vi "Run.vi"(8 "error in (no error)":errorcluster) -> (0 "error out":errorcluster)   [LabVIEW 2017, in "loggingModule.lvlib"]
uses:
  loggingModule.lvlib
  UEFGV/Type Def/UEFGV_States.ctl
  TypeDefs/LoopStates.ctl
  Queue/TypeDefs/queueFGVState.ctl
  ErrorMonitor/ErrorMonitor.lvlib
panel:
  out "stop":bool
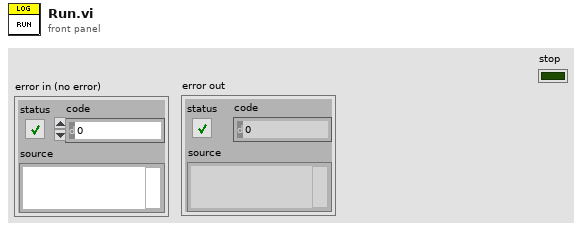
[diagram p1: front panel]
types:
  T1 = typedef "UEFGV_States.ctl" = enum16{"Create", "Get", "Destroy"}
  T2 = enum16{"open", "replace", "create", "open or create", "replace or create", "replace or create with confirmation"}
  T3 = typedef "LoopStates.ctl" = enum16{"start", "wait", "run", "end"}
  T4 = typedef "loggingModule.lvlib/queueFGVState.ctl" = enum16{"obtain", "enqueue low priority", "enqueue high priority", "dequeue", "release"}
  T5 = typedef "loggingModule.lvlib/message.ctl" = cluster{"calling module":string, "message":string, "data":variant}
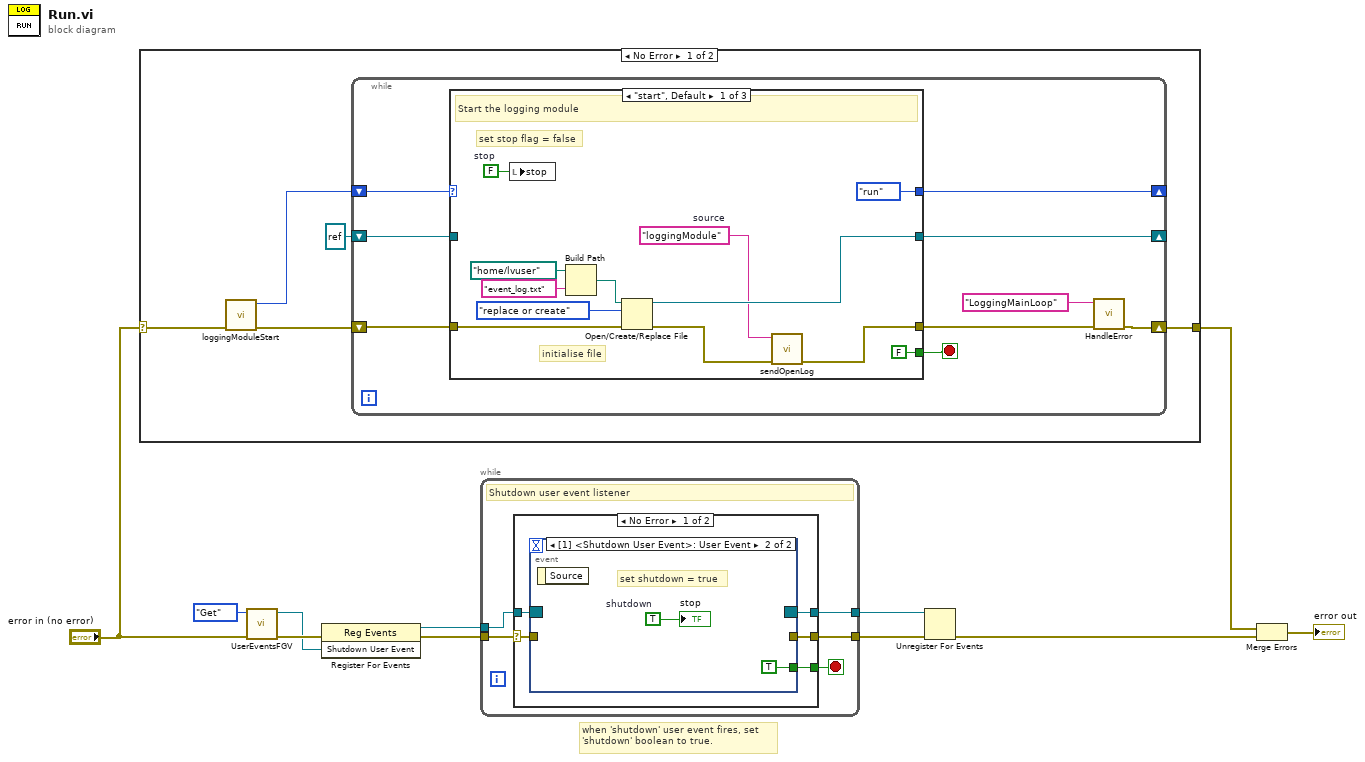
[diagram p0: block diagram]
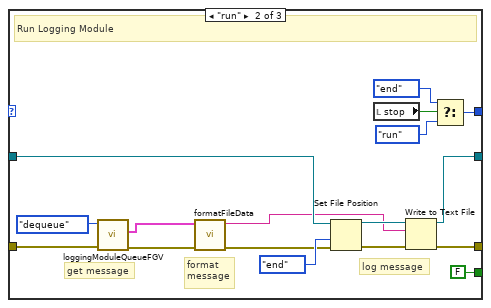
[diagram p2: hidden frame]
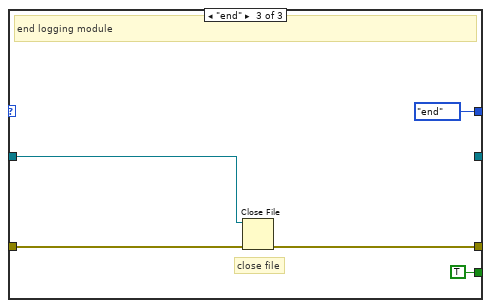
[diagram p3: hidden frame]
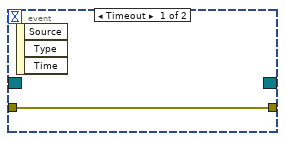
[diagram p5: hidden frame]
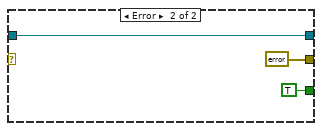
[diagram p6: hidden frame]
diagram:
  # "when 'shutdown' user event fires, set\n'shutdown' boolean to true."
  n1 = case shown="No Error" "error in (no error)" {
    selector: "error in (no error)" -> [w16 w60]
    tunnel: [w12 w60] -> w3
    frame No Error {
      n2 = call "loggingModuleStart.vi"("error in (no error)"=w16) -> ("error out"=w14:errorcluster, "message out"=w15:T3)  [unwired: 9 in]
      n3 = while {
        shift-right: [w23] -> _
        shift-left: w15 -> [w25]
        shift-right: [w17] -> w12
        shift-left: w14 -> [w22]
        shift-right: [w21] -> _
        shift-left: refnum<file> refnum ("refnum out") -> [w20]
        stop <- w24 stop-if-true
        n4 = case shown="\"start\", Default" w25 {
          tunnel: [FALSE FALSE TRUE] -> w24
          tunnel: [LoopStates."run" ("message out") w50 LoopStates."end" ("message out")] -> w23
          tunnel: w22 -> [w30 w49 w57]
          tunnel: [w27 w47 w56] -> w18
          tunnel: [w29 w44 _] -> w21
          tunnel: w20 -> [_ w45 w55]
          frame "start", Default {
            w26 = "loggingModule"  # source
            w35 = FALSE  # stop
            # "initialise file"
            # "set stop flag = false"
            # "Start the logging module"
            n5 = local write "stop"(w35) -> ()
            n6 = Build Path(base path=path "/home/lvuser", name or relative path="event_log.txt") -> (appended path=w32:path)
            n7 = Open/Create/Replace File(file path (use dialog)=w32, error in=w30, operation (0:open)=T2."replace or create") -> (refnum out=w29:refnum<file>, error out=w28:errorcluster)  [unwired: 3 in, 1 out]
            n8 = call "sendOpenLog.vi"("error in (no error)"=w28, "source"=w26) -> ("error out"=w27:errorcluster)  [unwired: 9 in]
          }
          frame "run" {
            # "log message"
            # "format\nmessage"
            # "get message"
            # "Run Logging Module"
            n9 = call "loggingModuleQueueFGV.vi"("error in (no error)"=w49, "command"=queueFGVState."dequeue") -> ("error out"=w40:errorcluster, "message out"=w41:T5)  [unwired: 8 in]
            n10 = call "formatFileData.vi"("error in (no error)"=w40, "message out"=w41) -> ("error out"=w39:errorcluster, "LogData"=w38:string)  [unwired: 8 in]
            n11 = Set File Position(refnum=w45, from (0:start)=enum16{"start", "end", "current"}."end", error in=w39) -> (refnum out=w46:refnum<file>, error out=w43:errorcluster)  [unwired: 1 in]
            n12 = local read "stop"() -> (w53:bool)
            n13 = Write to Text File(file (use dialog)=w46, text=w38, error in=w43) -> (refnum out=w44:refnum<file>, error out=w47:errorcluster)  [unwired: 1 in, 1 out]
            n14 = Select(t=LoopStates."end" ("message out"), s=w53, f=LoopStates."run" ("message out")) -> (s? t:f=w50:T3)
          }
          frame "end" {
            # "close file"
            # "end logging module"
            n15 = Close File(refnum=w55, error in=w57) -> (error out=w56:errorcluster)  [unwired: 1 out]
          }
        }
        n16 = call "HandleError.vi"("error in (no error)"=w18, "Source"="LoggingMainLoop") -> ("error out"=w17:errorcluster)  [unwired: 9 in]
      }
    }
    frame Error {
    }
  }
  n17 = call "UserEventsFGV.vi"("error in (no error)"="error in (no error)", "Command"=UEFGV_States."Get") -> ("error out"=w9:errorcluster, "Shutdown User Event"=w8:refnum<user-event>)  [unwired: 8 in]
  n18 = register-events(error in=w9, w8) -> (reference out=w11:refnum<event-registration>, error out=w6:errorcluster)  [unwired: 1 in]
  n19 = while {
    tunnel: w11 -> [w65]
    tunnel: [w64] -> w10
    tunnel: w6 -> [w62]
    tunnel: [w61] -> w7
    stop <- w63 stop-if-true
    # "Shutdown user event listener"
    n20 = case shown="No Error" w62 {
      selector: w62 -> [w67 _]
      tunnel: w65 -> [w70 w75]
      tunnel: [w69 w75] -> w64
      tunnel: [w68 TRUE] -> w63
      tunnel: [w66 errorcluster {"status"=FALSE, "code"=0, "source"=""} ("error out")] -> w61
      frame No Error {
        n21 = event shown="[1] <Shutdown User Event>: User Event" {
          selector: w70 -> [_ _]
          dyn-events: [_ _] -> w69
          timeout: _ -> [_ _]
          tunnel: w67 -> [w71 _]
          tunnel: [w71 _] -> w66
          tunnel: [_ TRUE] -> w68
          event Timeout {
            n22 = event-data() -> ()  [unwired: 1 in, 3 out]
          }
          event User Event {
            w72 = TRUE  # shutdown
            # "set shutdown = true"
            n23 = event-data() -> ()  [unwired: 1 in, 1 out]
            "stop" <- w72
          }
        }
      }
      frame Error {
      }
    }
  }
  n24 = Unregister For Events(event registration refnum=w10, error in=w7) -> (error out=w2:errorcluster)
  n25 = Merge Errors(w3, w2) -> (→"error out":errorcluster)
